vi "Write Origin.vi"(8 "error in (no error)":errorcluster, 10 "Origin":T1, 11 "Picture.lvclass in":refnum<class "Picture.lvclass">) -> (0 "error out":errorcluster, 3 "Picture.lvclass out":refnum<class "Picture.lvclass">)   [LabVIEW 2015, in "Picture.lvclass"]
uses:
  Picture.lvclass
  <vilib>/Utility/miscctls.llb/LVPointTypeDef.ctl
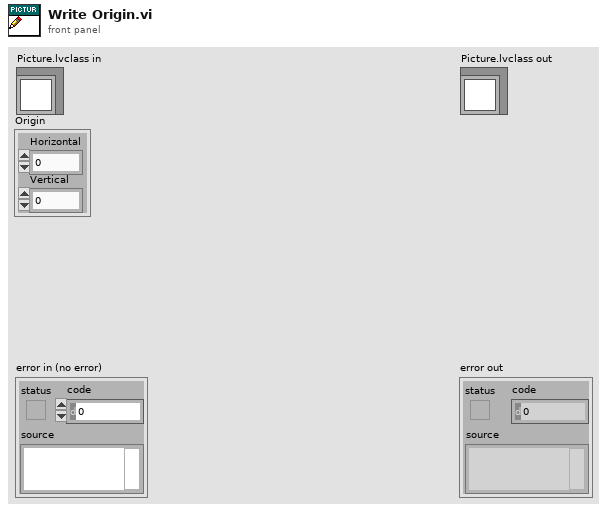
[diagram p1: front panel]
types:
  T1 = typedef "LVPointTypeDef.ctl" = cluster{"Horizontal":i16, "Vertical":i16}
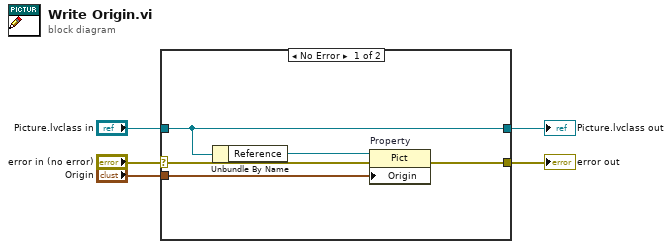
[diagram p0: block diagram]
diagram:
  n1 = case shown="No Error" "error in (no error)" {
    selector: "error in (no error)" -> [w6 w12]
    tunnel: [w10 w12] -> w4
    tunnel: [w8 w11] -> w2
    tunnel: "Picture.lvclass in" -> [w8 w11]
    tunnel: "Origin" -> [w9 _]
    frame No Error {
      n2 = Unbundle By Name(w8) -> ("Reference"=w7:refnum<vi>)
      n3 = property on="Property" class="Pict"(reference=w7, error in=w6, "Origin"=w9) -> (error out=w10:errorcluster)  [unwired: 1 out]
    }
    frame Error {
    }
  }
  "error out" <- w4
  "Picture.lvclass out" <- w2
